vi "fileIO_avg_speed_test.vi"() -> ()   [LabVIEW 2020]
uses:
  <vilib>/Utility/file.llb/Read Delimited Spreadsheet (string).vi
  <vilib>/Analysis/1siggen.llb/Ramp Pattern by Delta.vi
  <vilib>/Utility/file.llb/Write Delimited Spreadsheet (DBL).vi
  <vilib>/Analysis/NI_AALBase.lvlib
panel:
  out "auto 1000 m":dbl
  out "manual":dbl
  out "timestamp":dbl
  in  "out file path":path=path "C:/Users/Lenovo/Desktop/faszom.csv"
  out "time from 1000 m":dbl
  out "distance from 1000 m":dbl
  out "mean speed from 1000 m":dbl
  out "distance from manual pos":dbl
  out "XY Graph":cluster{timestamp[], dbl[]}[](graph)
  out "flag-timestamp array":cluster{"String":string, timestamp}[](array[cluster])
  out "time from timestamps":dbl format="%0.3f"
  out "true time from speed":dbl format="%0.3f"
  out "time from manual pos":dbl
  out "mean speed from speed":dbl format="%0.3f"
  out "mean speed from manual pos":dbl format="%0.3f"
  out "header out":T1
  in  "csv file path":path
  out "all rows":string[][](array[string])
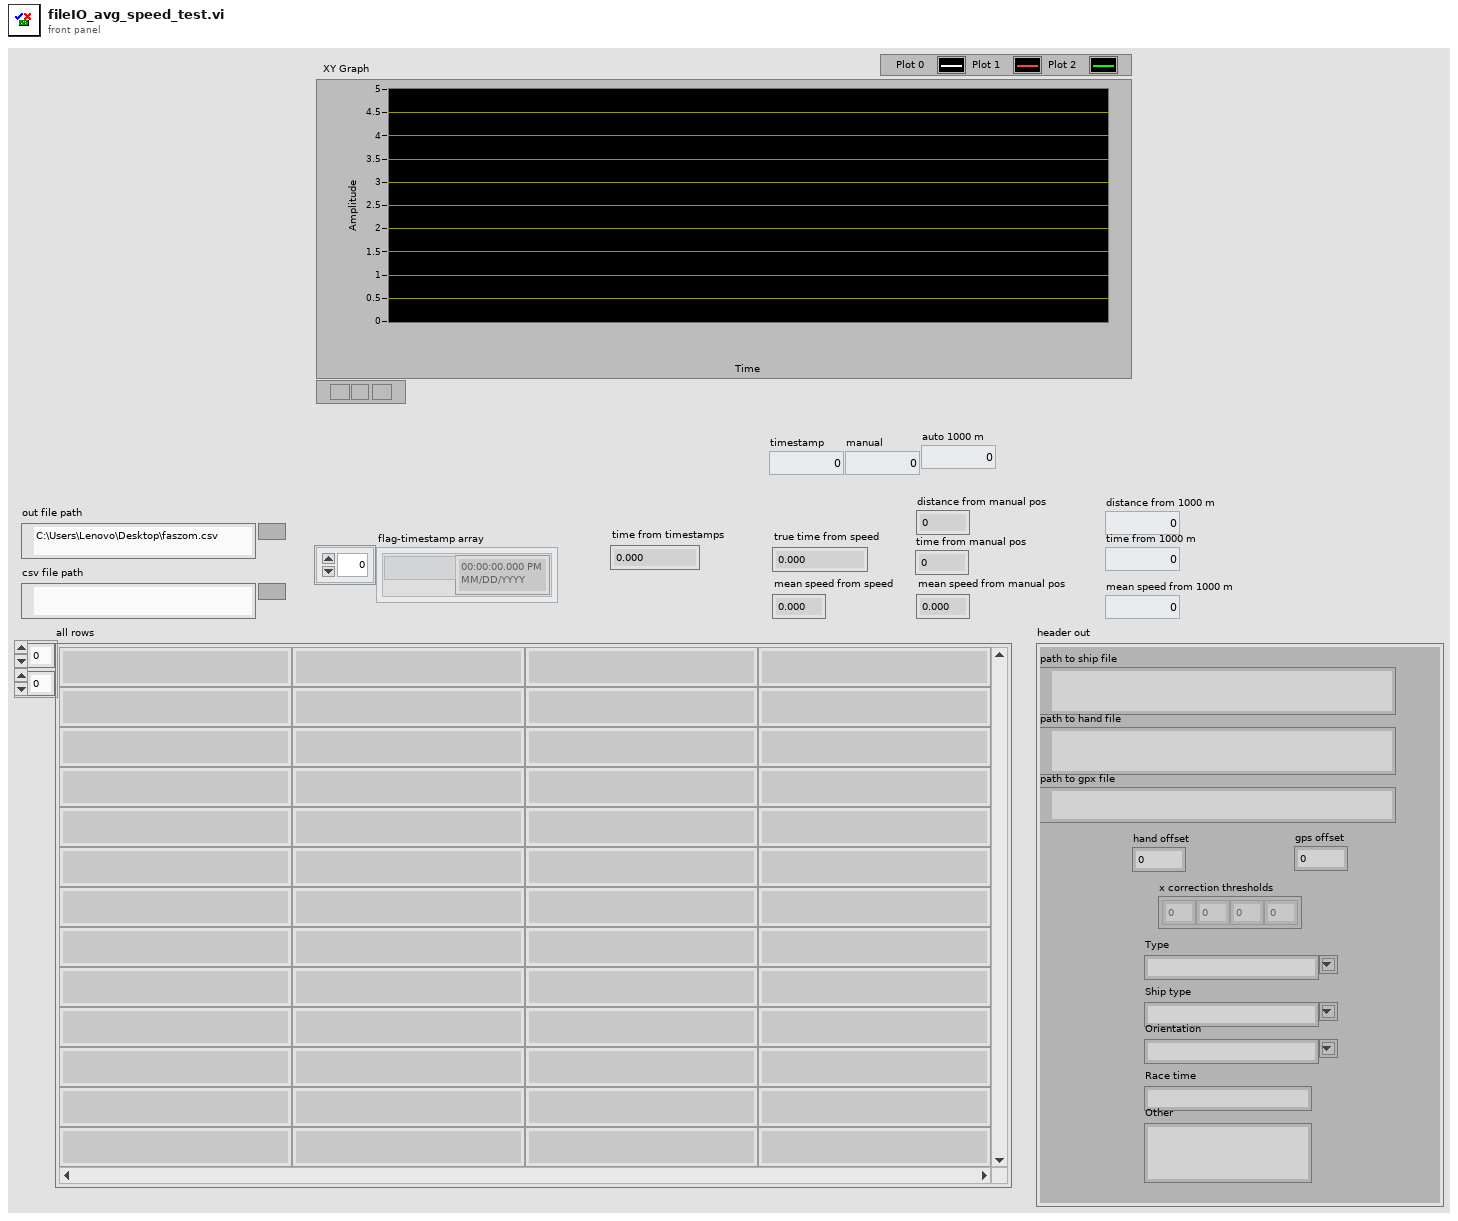
[diagram p1: front panel]
types:
  T1 = cluster{"path to ship file":path, "path to hand file":path, "path to gpx file":path, "hand offset":dbl, "gps offset":dbl, "x correction thresholds":i32[], "Type":string, "Ship type":string, "Orientation":string, "Race time":string, "Other":string}
  T2 = cluster{"Array":timestamp[], "Array":dbl[], "Array":dbl[]}
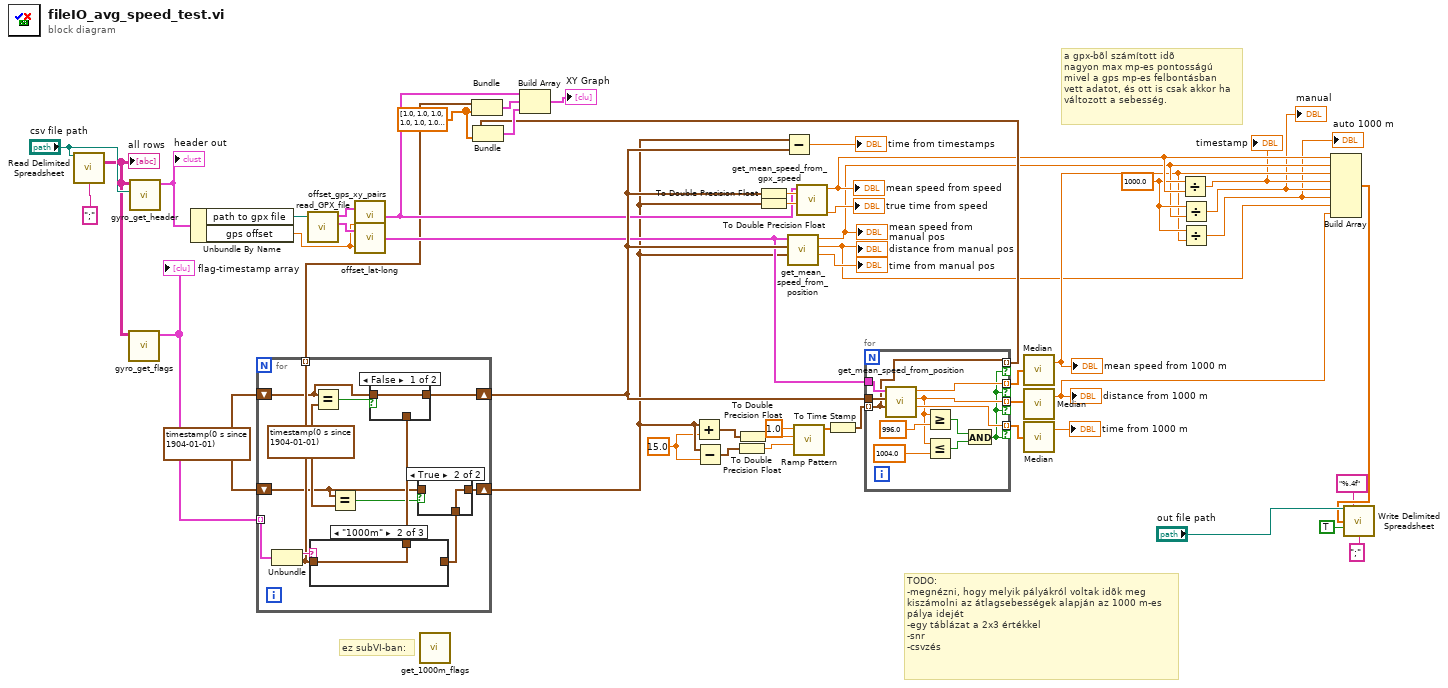
[diagram p0: block diagram]
diagram:
  w8 = 1000.0 ("x")
  w28 = 15.0 ("delta")
  w21 = dbl[] [1.0, 1.0, 1.0, 1.0, 1.0, 1.0, 1.0, 1.0, 1.0, 1.0, 1.0, 1.0, 1.0, 1.0, 1.0, 1.0, 1.0, 1.0, 1.0, 1.0]
  w38 = timestamp(0 s since 1904-01-01)
  # "ez subVI-ban:"
  # "a gpx-bõl számított idõ\nnagyon max mp-es pontosságú\nmivel a gps mp-es felbontásban\nvett adatot, és ott is csak akkor ha\nváltozott a sebesség."
  # "TODO: \n-megnézni, hogy melyik pályákról voltak idõk meg\nkiszámolni az átlagsebességek alapján az 1000 m-es\npálya idejét\n-egy táblázat a 2x3 értékkel\n-snr\n-csvzés"
  n1 = call-poly <vilib>:"Read Delimited Spreadsheet.vi"("file path (dialog if empty)"="csv file path", "delimiter (\\t)"=";" ("delimiter (\\t)")) -> ("all rows"=w47:string[][])  [unwired: 8 in, 5 out]
  "all rows" <- w47
  n2 = call "gyro_get_flags.vi"("all rows"=w47) -> ("flag-timestamp array"=w45:cluster{"String":string, timestamp}[])  [unwired: 10 in]
  "flag-timestamp array" <- w45
  n3 = call "gyro_get_header.vi"("csv path"="csv file path", "all rows"=w47) -> ("header out"=w49:T1)  [unwired: 9 in]
  "header out" <- w49
  n4 = Unbundle By Name(w49) -> ("path to gpx file"=w48:path, "gps offset"=w36:dbl)
  n5 = for {
    shift-right: [w58] -> w39
    shift-left: w38 -> [w57]
    shift-right: [w55] -> w29
    shift-left: w38 -> [w52]
    tunnel: w45 -> [w63] mode=indexing
    tunnel: [w61] -> w31 mode=indexing
    w53 = timestamp(0 s since 1904-01-01)
    n6 = Unbundle(w63) -> ("String"=w62:string, w61:timestamp)
    n7 = case shown="\"1000m\"" w62 {
      tunnel: w61 -> [_ w68 w69]
      tunnel: [_ w68 _] -> w59
      tunnel: [_ _ w69] -> w56
      frame Default {
      }
      frame "1000m" {
      }
      frame "1000m_end" {
      }
    }
    n8 = Equal?(x=w57, y=w53) -> (x = y?=w60:bool)
    n9 = Equal?(x=w52, y=w53) -> (x = y?=w54:bool)
    n10 = case shown="False" w60 {
      tunnel: w59 -> [_ w67]
      tunnel: [w66 w67] -> w58
      tunnel: w57 -> [w66 _]
      frame False {
      }
      frame True {
      }
    }
    n11 = case shown="True" w54 {
      tunnel: w56 -> [_ w65]
      tunnel: [w64 w65] -> w55
      tunnel: w52 -> [w64 _]
      frame False {
      }
      frame True {
      }
    }
  }
  n12 = call "read_GPX_file.vi"("GPX File Path"=w48) -> ("lat/lon position"=w46:cluster{timestamp[], dbl[], dbl[]}, "XY Speed data"=w37:cluster{timestamp[], dbl[]})  [unwired: 3 in, 2 out]
  n13 = call "offset_gps_xy_pairs.vi"("offset"=w36, "XY data"=w37) -> ("XY data"=w34:cluster{timestamp[], dbl[]})
  n14 = call "offset_lat-long.vi"("gps offset"=w36, "lat/lon position"=w46) -> ("Cluster"=w33:T2)
  n15 = call "get_1000m_flags.vi"() -> ()  [unwired: 2 in, 2 out]
  n16 = Bundle(w31, w21) -> (w32:cluster{timestamp[], dbl[]})  [unwired: 1 in]
  n17 = Add(x=w29, y=w28) -> (x+y=w26:timestamp)
  n18 = Subtract(x=w29, y=w28) -> (x-y=w25:timestamp)
  n19 = To Double Precision Float(number=w25) -> (double precision float=w24:dbl)
  n20 = To Double Precision Float(number=w26) -> (double precision float=w27:dbl)
  n21 = To Double Precision Float(number=w39) -> (double precision float=w40:dbl)
  n22 = To Double Precision Float(number=w29) -> (double precision float=w41:dbl)
  n23 = Subtract(x=w29, y=w39) -> (x-y=→"time from timestamps":dbl)
  n24 = call "get_mean_speed_from_position.vi"("end"=w29, "start"=w39, "lat/lon position"=w33) -> ("dt [s]"=→"time from manual pos":dbl, "distance [m]"=w2:dbl, "mean speed [m/s]"=w7:dbl)  [unwired: 6 in]
  "mean speed from manual pos" <- w7
  "distance from manual pos" <- w2
  n25 = call-poly <vilib>:"Ramp Pattern.vi"("start"=w24, "end"=w27, "delta"=1.0) -> ("Ramp Pattern"=w23:dbl[])  [unwired: 6 in, 2 out]
  n26 = call "get_mean_speed_from_gpx_speed.vi"("to"=w41, "from"=w40, "speed"=w34) -> ("true dt"=→"true time from speed":dbl, "mean"=w9:dbl)  [unwired: 5 in, 2 out]
  "mean speed from speed" <- w9
  n27 = To Time Stamp(1:w23) -> (0:w20:timestamp[])
  n28 = for {
    tunnel: w39 -> [w80]
    tunnel: w33 -> [w79]
    tunnel: w20 -> [w71] mode=indexing
    tunnel: [w78] -> w18 mode=indexing if=w70
    tunnel: [w73] -> w17 mode=indexing if=w70
    tunnel: [w77] -> w16 mode=indexing if=w70
    tunnel: [w71] -> w19 mode=indexing if=w70
    n29 = call "get_mean_speed_from_position.vi"("end"=w71, "start"=w80, "lat/lon position"=w79) -> ("dt [s]"=w77:dbl, "distance [m]"=w73:dbl, "mean speed [m/s]"=w78:dbl)  [unwired: 6 in]
    n30 = Greater Or Equal?(x=w73, y=996.0) -> (x >= y?=w76:bool)
    n31 = Less Or Equal?(x=w73, y=1004.0) -> (x <= y?=w72:bool)
    n32 = And(x=w76, y=w72) -> (x .and. y?=w70:bool)
  }
  n33 = Bundle(w19, w21) -> (w22:cluster{timestamp[], dbl[]})  [unwired: 1 in]
  n34 = Build Array(w34, w32, w22) -> (→"XY Graph":cluster{timestamp[], dbl[]}[])
  n35 = call <vilib>:"Median.vi"("X"=w18) -> ("median"=w6:dbl)  [unwired: 1 out]
  "mean speed from 1000 m" <- w6
  n36 = call <vilib>:"Median.vi"("X"=w17) -> ("median"=w1:dbl)  [unwired: 1 out]
  "distance from 1000 m" <- w1
  n37 = call <vilib>:"Median.vi"("X"=w16) -> ("median"=→"time from 1000 m":dbl)  [unwired: 1 out]
  n38 = Divide(x=w8, y=w9) -> (x/y=w5:dbl)
  "timestamp" <- w5
  n39 = Divide(x=w8, y=w7) -> (x/y=w4:dbl)
  "manual" <- w4
  n40 = Divide(x=w8, y=w6) -> (x/y=w3:dbl)
  "auto 1000 m" <- w3
  n41 = Build Array(w9, w7, w6, w5, w4, w3, w2, w1) -> (w12:dbl[])
  n42 = call-poly <vilib>:"Write Delimited Spreadsheet.vi"("file path (dialog if empty)"="out file path", "format (%.3f)"="%.4f", "1D data"=w12, "append to file? (new file:F)"=TRUE, "delimiter (\\t)"=";" ("delimiter (\\t)")) -> ()  [unwired: 9 in, 2 out]
